vi "Class - ResultCntr.Init.vi"(8 "error in (no error)":errorcluster, 11 "Class - ResultCntr in":refnum<class "Class - ResultCntr.lvclass">) -> (0 "error out":errorcluster, 3 "Class - ResultCntr out":refnum<class "Class - ResultCntr.lvclass">)   [LabVIEW 2024, in "EQMF.lvlib" / "Results.lvlib" / "Class - ResultCntr.lvclass"]
uses:
  Class - ResultCntr.lvclass
  Class - ResultCntr.lvclass/Class - ResultCntr.ctl
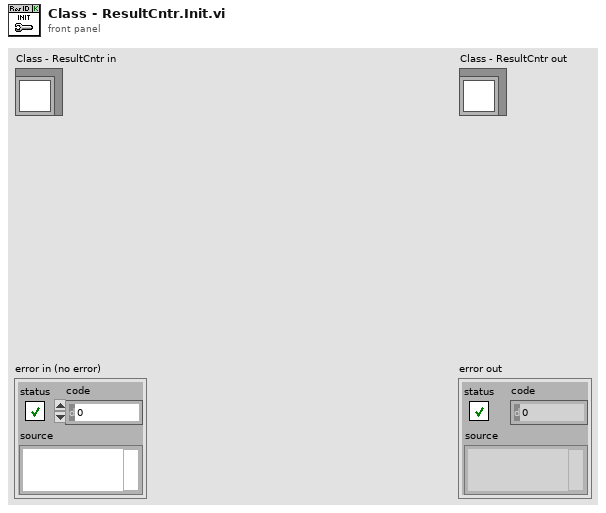
[diagram p1: front panel]
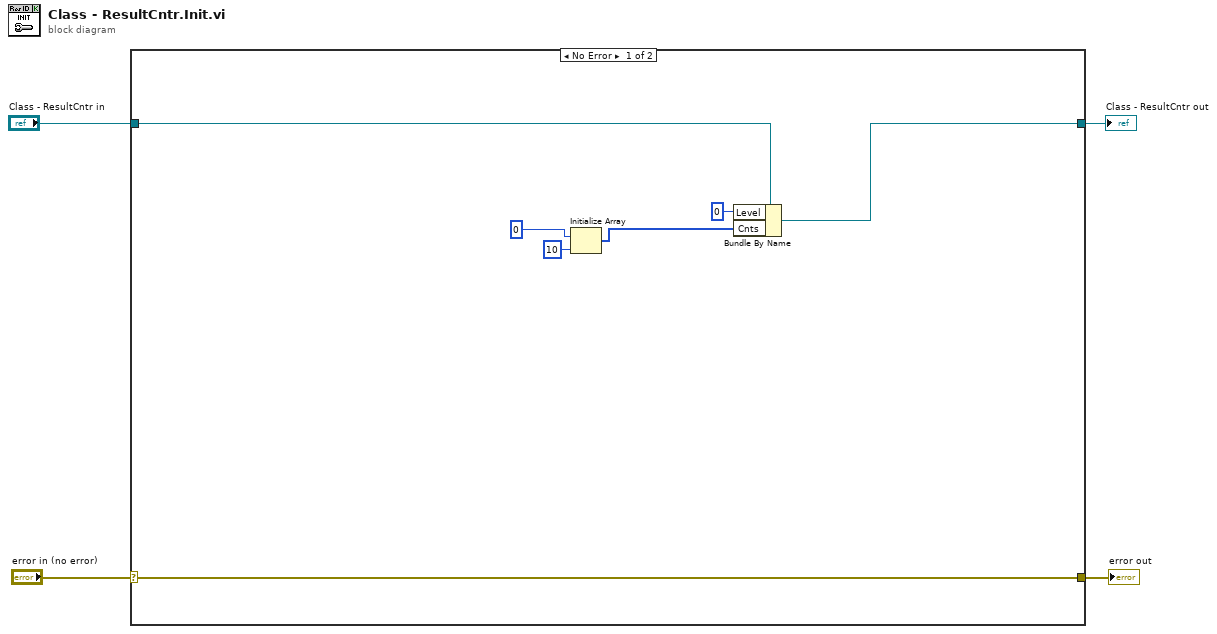
[diagram p0: block diagram]
diagram:
  n1 = case shown="No Error" "error in (no error)" {
    selector: "error in (no error)" -> [w11 w13]
    tunnel: [w11 w13] -> w3
    tunnel: [w9 w12] -> w1
    tunnel: "Class - ResultCntr in" -> [w10 w12]
    frame No Error {
      n2 = Initialize Array(0 ("Level"), 10 ("dimension size")) -> (w5:i32[])
      n3 = Bundle By Name(cluster=w10, "Level"=0, "Cnts"=w5) -> (w9:refnum<class "Class - ResultCntr.lvclass">)
    }
    frame Error {
    }
  }
  "error out" <- w3
  "Class - ResultCntr out" <- w1
